vi "Fit.vi"(7 "Type X":T1(ring), 8 "error in (no error)":errorcluster caption="entrée d'erreur (pas d'erreur)", 9 "y":string[][](array[string]), 10 "X":string[][](array[string]), 11 "SparseRandomProjection.lvclass":refnum<class "SparseRandomProjection.lvclass">) -> (0 "error out":errorcluster caption="sortie d'erreur", 2 "String Data":string, 3 "SparseRandomProjection.lvclass":refnum<class "SparseRandomProjection.lvclass">)   [LabVIEW 2020, in "SparseRandomProjection.lvclass"]
doc: "Generate a sparse random projection matrix\n\nReturns : \n\n- String : OK"
uses:
  SparseRandomProjection.lvclass
  SparseRandomProjection.lvclass/SparseRandomProjection.ctl
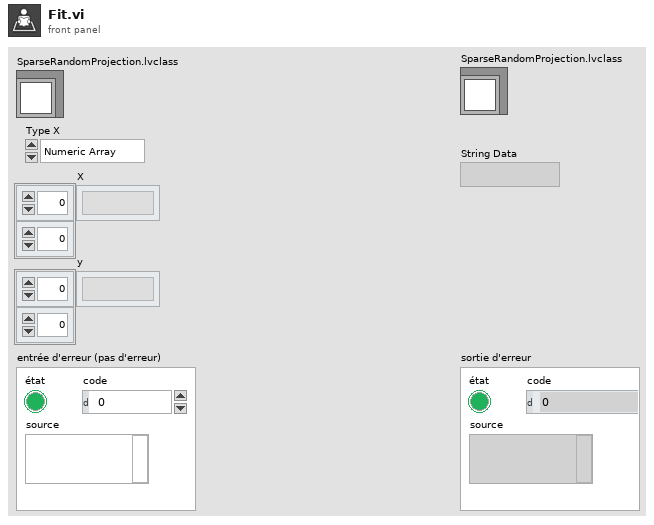
[diagram p1: front panel]
types:
  T1 = enum16{"Numeric Array", "String Array", "Sparse"}
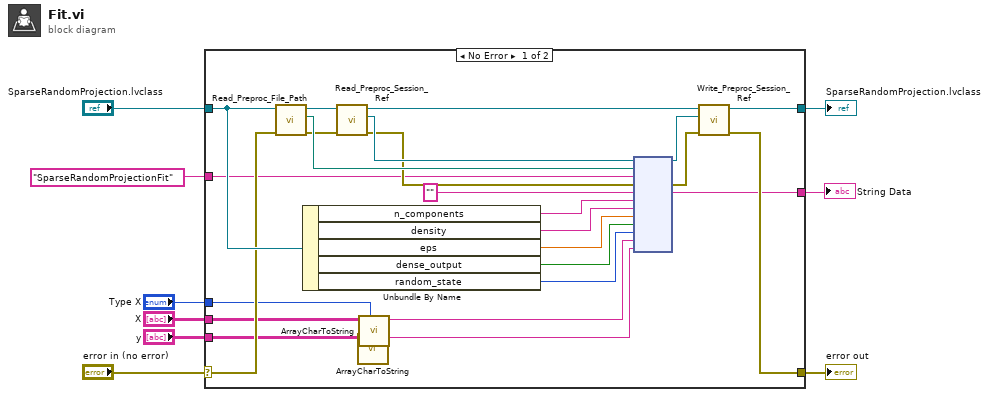
[diagram p0: block diagram]
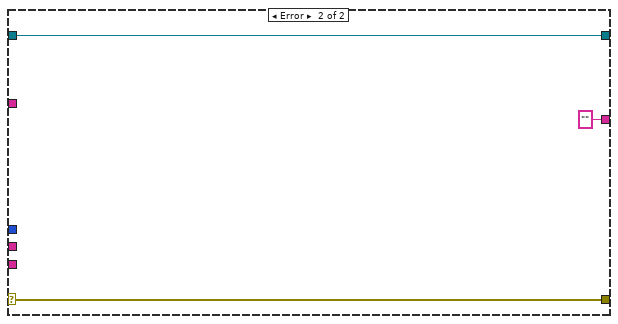
[diagram p2: hidden frame]
diagram:
  n1 = case shown="No Error" "error in (no error)" {
    selector: "error in (no error)" -> [w23 w37]
    tunnel: [w22 w37] -> w8
    tunnel: [w24 w36] -> w6
    tunnel: "SparseRandomProjection.lvclass" -> [w25 w36]
    tunnel: "SparseRandomProjectionFit" ("Fonction") -> [w21 _]
    tunnel: [w20 ""] -> w4
    tunnel: "X" -> [w14 _]
    tunnel: "y" -> [w12 _]
    tunnel: "Type X" -> [w10 _]
    frame No Error {
      n2 = call-dynamic "Read_Preproc_File_Path.vi"("error in (no error)"=w23, "Python in"=w25) -> ("error out"=w29:errorcluster, "File_Path"=w32:path, "Python out"=w34:refnum<class "SparseRandomProjection.lvclass">)  [unwired: 7 in]
      n3 = Unbundle By Name(w25) -> ("n_components"=w19:string, "density"=w18:string, "eps"=w17:dbl, "dense_output"=w16:bool, "random_state"=w15:i32)
      n4 = call-dynamic "Read_Preproc_Session_Ref.vi"("error in (no error)"=w29, "Python in"=w34) -> ("error out"=w30:errorcluster, "Session_ref"=w31:refnum<k35>, "Python out"=w33:refnum<class "SparseRandomProjection.lvclass">)  [unwired: 7 in]
      n5 = call "ArrayCharToString.vi"("TAB"=w12) -> ("Instruction"=w11:string)  [unwired: 10 in]
      n6 = call "ArrayCharToString.vi"("Type"=w10, "TAB"=w14) -> ("Instruction"=w13:string)  [unwired: 9 in]
      n7 = node(w31, w32, w21, w30, "", w19, w18, w17, w16, w15, w13, w11) -> (w26:refnum<k35>, w28:errorcluster, w20:string)  [unwired: 7 in, 2 out]
      n8 = call-dynamic "Write_Preproc_Session_Ref.vi"("error in (no error)"=w28, "Session_ref"=w26, "Python in"=w33) -> ("error out"=w22:errorcluster, "Python out"=w24:refnum<class "SparseRandomProjection.lvclass">)  [unwired: 7 in]
    }
    frame Error {
    }
  }
  "error out" <- w8
  "SparseRandomProjection.lvclass" <- w6
  "String Data" <- w4
